vi "Test Client.vi"() -> ()   [LabVIEW 2016, in "Instrument.Example.lvclass"]
uses:
  Instrument.Example.lvclass
  <userlib>/LevyLab/Levylab Instruments/SMOs/RemoteControl/Typedefs/Message--Cluster.ctl
  <userlib>/_OpenG.lib/numeric/numeric.llb/Random Number Within Range - DBL__ogtk.vi
  <userlib>/LevyLab/Levylab Instruments/SMOs/RemoteControl/RemoteControl.lvclass
panel:
  out "Numeric":i32
  in  "stop":bool
  out "Waveform Chart":u32(graph)
  out "error out":errorcluster
  out "execution time (ms)":u32
  out "Message Received":T1
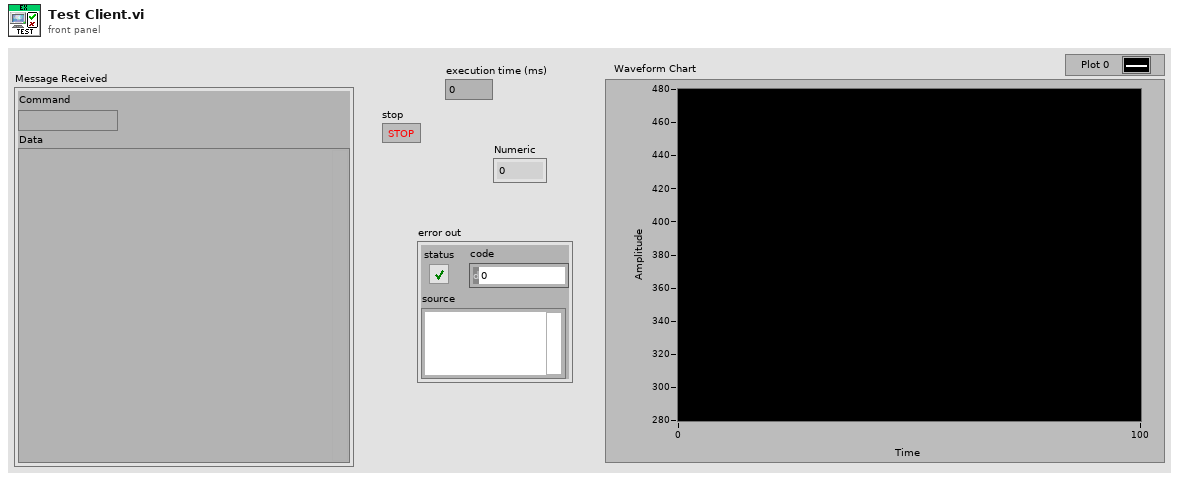
[diagram p1: front panel]
types:
  T1 = typedef "RemoteControl.lvclass/Message--Cluster.ctl" = cluster{"Command":string, "Data":variant}
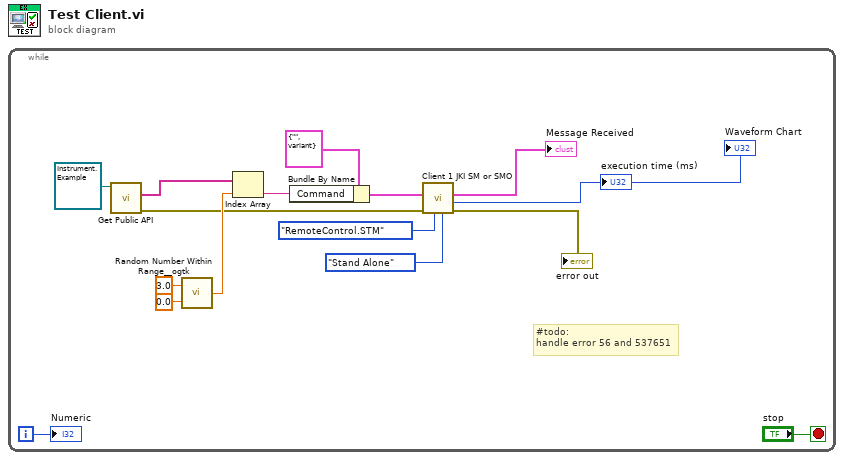
[diagram p0: block diagram]
diagram:
  n1 = while {
    i -> [w6]
    stop <- "stop" stop-if-true
    # "#todo:\nhandle error 56 and 537651"
    n2 = call-dynamic "Get Public API.vi"("Instrument.Example In"=refnum<class "Instrument.Example.lvclass"> refnum ("Instrument.SR7270 in")) -> ("error out"=w2:errorcluster, "Commands"=w1:string[])  [unwired: 8 in, 1 out]
    n3 = call-poly <userlib>:"Random Number Within Range__ogtk.vi"("High"=3.0, "Low"=0.0) -> ("Random Number"=w11:dbl)  [unwired: 3 in]
    n4 = Index Array(array=w1, index=w11) -> (element=w14:string)
    n5 = Bundle By Name(cluster=T1 {"Command"="", "Data"=variant} ("Message to Send"), "Command"=w14) -> (w15:T1)
    n6 = call <userlib>:"Client 1 JKI SM or SMO.vi"("Enum 2"=enum16{"SMO", "Stand Alone"}."Stand Alone", "Enum"=enum16{"RemoteControl", "RemoteControl.STM"}."RemoteControl.STM", "error in (no error)"=w2, "Message to Send"=w15) -> ("error out"=→"error out":errorcluster, "execution time (ms)"=→"execution time (ms)" →"Waveform Chart":u32, "Message Received"=→"Message Received":T1)  [unwired: 5 in]
    "Numeric" <- w6
  }
